vi "Update Plugin to Abort.vi"(8 "error in (no error)":errorcluster, 11 "CIF_UI in":refnum<class "CIF_UI.lvclass">) -> (0 "error out":errorcluster, 3 "CIF_UI out":refnum<class "CIF_UI.lvclass">)   [LabVIEW 2021, in "CIF_UI.lvclass"]
uses:
  CIF_UI.lvclass
  CIF_UI.lvclass/CIF_UI.ctl
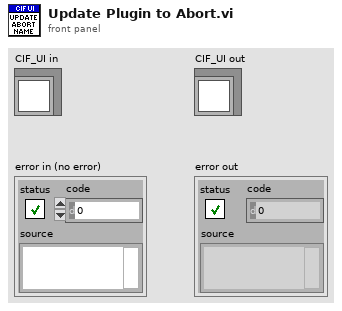
[diagram p1: front panel]
types:
  T1 = typedef "CIF_UI.lvclass/Plugin Connection Map.ctl" = map{string, T2}
  T2 = typedef "CIF_UI.lvclass/Plugin Connections.ctl" = cluster{"gRPC ID":T3, "Plugin info":T4}
  T3 = typedef "grpc-lvsupport-release.lvlib/grpcId.ctl" = u64
  T4 = typedef "CIF_Manager_client.lvlib/cif_manager_PluginInfo.ctl" = cluster{"plugin_name":string, "plugin_type":string, "grpc_port":i32, "plugin_version":T5, "status":T6}
  T5 = typedef "CIF_Manager_client.lvlib/cif_manager_PluginVersion.ctl" = cluster{"major_version":i32, "minor_version":i32, "fix_version":i32, "build_version":i32}
  T6 = typedef "CIF_Manager_client.lvlib/cif_plugincore_StatusData.ctl" = cluster{"state":T7, "timing_statistics":T8, "fifo_statistics":T10, "error":T11, "monitor_doubles":T12, "monitor_u64s":T13, "monitor_i64s":T14}
  T7 = typedef "CIF_Manager_client.lvlib/cif_plugincore_StatusData_State.ctl" = enum32{"NULL", "CREATING", "LISTENING", "RUNNING", "CLEANINGUP", "DESTROYING"}
  T8 = typedef "CIF_Manager_client.lvlib/cif_plugincore_TimingStatistics.ctl" = cluster{"period":T9, "wake_error":T9, "execute":T9, "housekeep":T9, "idle":T9}
  T9 = typedef "CIF_Manager_client.lvlib/cif_plugincore_TimingStatsBasic.ctl" = cluster{"max":i32, "min":i32}
  T10 = typedef "CIF_Manager_client.lvlib/cif_plugincore_FifoStatistics.ctl" = cluster{"from_t0":T9, "from_previous_plugin":T9, "output_error":T9}
  T11 = typedef "CIF_Manager_client.lvlib/cif_plugincore_Error.ctl" = cluster{"status":bool, "code":i32}
  T12 = typedef "CIF_Manager_client.lvlib/cif_plugincore_MonitorDoubles.ctl" = cluster{"double_1":dbl, "double_2":dbl, "double_3":dbl, "double_4":dbl}
  T13 = typedef "CIF_Manager_client.lvlib/cif_plugincore_MonitorU64.ctl" = cluster{"u64_1":u64, "u64_2":u64, "u64_3":u64, "u64_4":u64}
  T14 = typedef "CIF_Manager_client.lvlib/cif_plugincore_MonitorI64.ctl" = cluster{"i64_1":i64, "i64_2":i64, "i64_3":i64, "i64_4":i64}
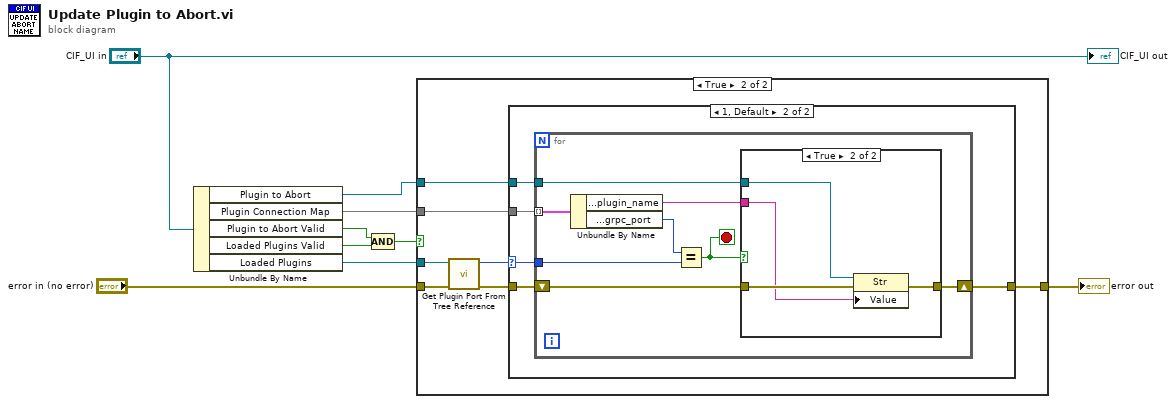
[diagram p0: block diagram]
diagram:
  n1 = Unbundle By Name("CIF_UI in") -> ("Plugin to Abort"=w1:refnum<vi>, "Plugin Connection Map"=w6:T1, "Plugin to Abort Valid"=w2:bool, "Loaded Plugins Valid"=w3:bool, "Loaded Plugins"=w9:refnum<vi>)
  n2 = Compound Arithmetic op=AND(w2, w3) -> (w8:bool)
  n3 = case shown="True" w8 {
    tunnel: w6 -> [_ w17]
    tunnel: "error in (no error)" -> [w10 w16]
    tunnel: w1 -> [_ w15]
    tunnel: w9 -> [_ w14]
    tunnel: [w10 w11] -> w7
    frame False {
    }
    frame True {
      n4 = call "Get Plugin Port From Tree Reference.vi"("error in (no error)"=w16, "Loaded Plugins"=w14) -> ("error out"=w13:errorcluster, "Plugin port"=w12:i32)  [unwired: 8 in]
      n5 = case shown="1, Default" w12 {
        selector: w12 -> [_ w20]
        tunnel: w17 -> [_ w23]
        tunnel: w15 -> [_ w22]
        tunnel: w13 -> [w18 w21]
        tunnel: [w18 w19] -> w11
        frame 0 {
        }
        frame 1, Default {
          n6 = for {
            tunnel: w23 -> [w31] mode=indexing
            tunnel: w20 -> [w30]
            tunnel: w22 -> [w26]
            shift-right: [w24] -> w19
            shift-left: w21 -> [w25]
            stop <- w28 stop-if-true
            n7 = Unbundle By Name(w31) -> ("Plugin Connections.Plugin info.plugin_name"=w27:string, "Plugin Connections.Plugin info.grpc_port"=w29:i32)
            n8 = Equal?(x=w29, y=w30) -> (x = y?=w28:bool)
            n9 = case shown="True" w28 {
              tunnel: w27 -> [_ w34]
              tunnel: w26 -> [_ w35]
              tunnel: w25 -> [w32 w36]
              tunnel: [w32 w33] -> w24
              frame False {
              }
              frame True {
                n10 = property class="Str"(reference=w35, error in=w36, "Value"=w34) -> (error out=w33:errorcluster)  [unwired: 1 out]
              }
            }
          }
        }
      }
    }
  }
  "error out" <- w7
  "CIF_UI out" <- "CIF_UI in"
